vi "Compute HR from Peaks.vi"(0 "Peak Locations In":dbl[](array[numeric]), 1 "Error In":errorcluster, 5 "Tolerance Fraction":dbl, 7 "Reference Lag from AutoCorrelation":dbl, 9 "Min Lag Index":dbl, 11 "Max Lag Index":dbl, 12 "dt":dbl) -> (3 "Keep This Lag?":bool, 4 "Filtered Lag Arrray":dbl[](array[numeric]), 6 "Periods (s)":dbl[](array[numeric]), 8 "Raw Lag Array":dbl[](array[numeric]), 10 "HR (bpm)":dbl, 13 "enough lags?":bool, 14 "valid HR?":bool, 15 "Error Out":errorcluster)   [LabVIEW 2025]
uses:
  <vilib>/Analysis/NI_AALBase.lvlib
panel:
  out "Matches Best Lag?":bool
  out "Lag in Physiologic Range?":bool
  out "Upper Bound":dbl
  out "Lower Bound":dbl
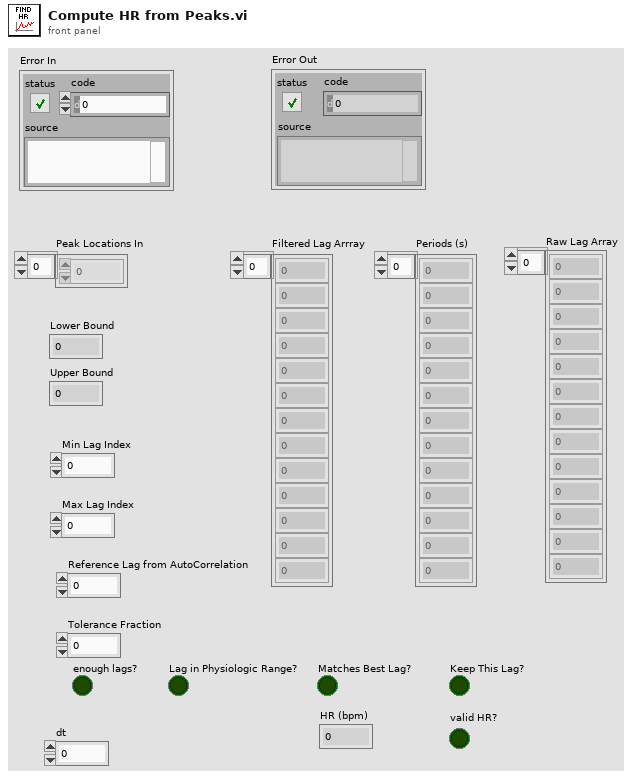
[diagram p1: front panel]
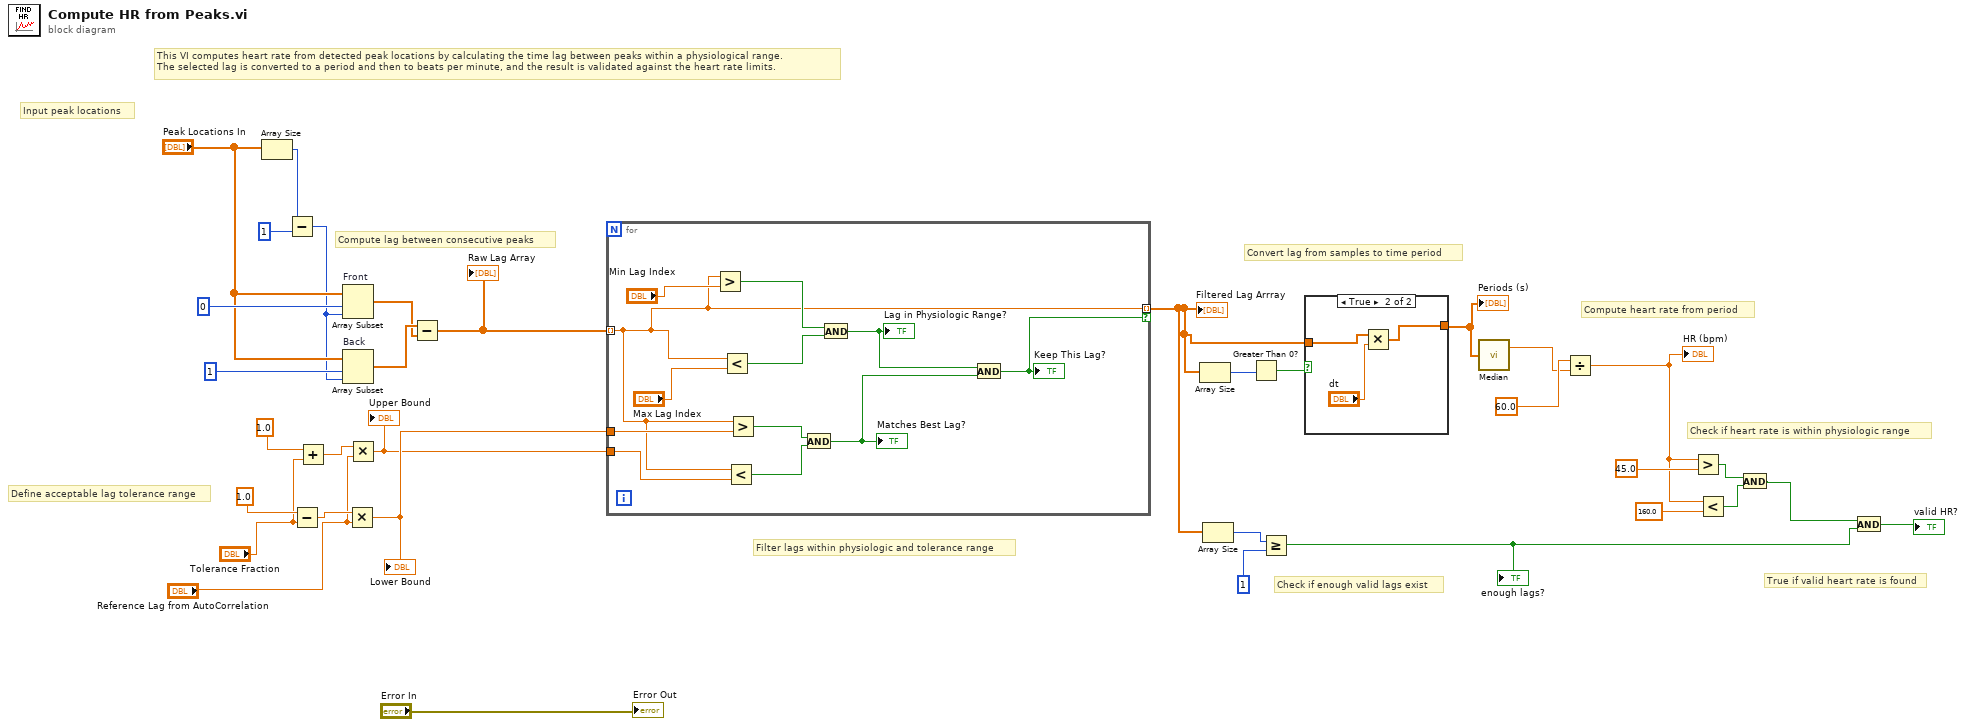
[diagram p0: block diagram]
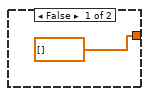
[diagram p2: hidden frame]
diagram:
  # "True if valid heart rate is found"
  # "Check if heart rate is within physiologic range"
  # "Compute heart rate from period"
  # "Convert lag from samples to time period"
  # "Check if enough valid lags exist"
  # "Filter lags within physiologic and tolerance range"
  # "Define acceptable lag tolerance range"
  # "Compute lag between consecutive peaks"
  # "Input peak locations"
  # "This VI computes heart rate from detected peak locations by calculating the time lag between peaks within a physiological range. \nThe selected lag is converted to a period and then to beats per minute, and the result is validated against the heart rate limits."
  n1 = Array Size(array="Peak Locations In") -> (size(s)=w21:i32)
  n2 = Subtract(x=w21, y=1) -> (x-y=w19:i32)
  n3 = Subtract(x=1.0, y="Tolerance Fraction") -> (x-y=w17:dbl)
  n4 = Add(x=1.0, y="Tolerance Fraction") -> (x+y=w14:dbl)
  n5 = Array Subset "Front"(array="Peak Locations In", index=0, length=w19) -> (w22:dbl[])
  n6 = Array Subset "Back"(array="Peak Locations In", index=1, length=w19) -> (w23:dbl[])
  n7 = Multiply(x=w17, y="Reference Lag from AutoCorrelation") -> (x*y=w11:dbl)
  "Lower Bound" <- w11
  n8 = Multiply(x=w14, y="Reference Lag from AutoCorrelation") -> (x*y=w10:dbl)
  "Upper Bound" <- w10
  n9 = Subtract(x=w23, y=w22) -> (x-y=w12:dbl[])
  "Raw Lag Array" <- w12
  n10 = for {
    tunnel: w12 -> [w36] mode=indexing
    tunnel: w11 -> [w44]
    tunnel: w10 -> [w43]
    tunnel: [w36] -> w2 mode=indexing if=w35
    n11 = Greater?(x=w36, y="Min Lag Index") -> (0:w42:bool)
    n12 = Less?(x=w36, y="Max Lag Index") -> (x < y?=w41:bool)
    n13 = Less?(x=w36, y=w43) -> (x < y?=w39:bool)
    n14 = Greater?(x=w36, y=w44) -> (0:w40:bool)
    n15 = And(x=w40, y=w39) -> (x .and. y?=w37:bool)
    "Matches Best Lag?" <- w37
    n16 = And(x=w42, y=w41) -> (x .and. y?=w38:bool)
    "Lag in Physiologic Range?" <- w38
    n17 = And(x=w38, y=w37) -> (x .and. y?=w35:bool)
    "Keep This Lag?" <- w35
  }
  "Filtered Lag Arrray" <- w2
  n18 = Array Size(array=w2) -> (size(s)=w4:i32)
  n19 = Array Size(array=w2) -> (size(s)=w33:i32)
  n20 = Greater Than 0?(x=w4) -> (x > 0?=w3:bool)
  n21 = Greater Or Equal?(x=w33, y=1) -> (x >= y?=w6:bool)
  "enough lags?" <- w6
  n22 = case shown="True" w3 {
    tunnel: w2 -> [_ w50]
    tunnel: [dbl[] [] w49] -> w1
    frame False {
    }
    frame True {
      n23 = Multiply(x=w50, y="dt") -> (x*y=w49:dbl[])
    }
  }
  "Periods (s)" <- w1
  n24 = call <vilib>:"Median.vi"("X"=w1) -> ("median"=w9:dbl)  [unwired: 1 out]
  n25 = Divide(x=60.0, y=w9) -> (x/y=w27:dbl)
  "HR (bpm)" <- w27
  n26 = Greater?(x=w27, y=45.0) -> (0:w30:bool)
  n27 = Less?(x=w27, y=160.0) -> (x < y?=w29:bool)
  n28 = And(x=w30, y=w29) -> (x .and. y?=w7:bool)
  n29 = And(x=w7, y=w6) -> (x .and. y?=→"valid HR?":bool)
  "Error Out" <- "Error In"
